vi "Keithley 2600 Series Merge.vi"() -> ()   [LabVIEW 2017]
doc: "This example shows how to create, run a script and query the script output data."
uses:
  <vilib>/Utility/file.llb/Write Delimited Spreadsheet (string).vi
  <instrlib>/Keithley 2600 Series/Keithley 2600 Series.lvlib
panel:
  in  "Yes":bool
  out "Continue":bool
  out "PCE(a.u.)":dbl
  in  "Pin(W/cm^2)":dbl=0.1
  out "FF(a.u.)":dbl
  out "Jsc(A/cm^2)":dbl
  in  "Area(cm^2)":dbl=0.085
  out "Ioc(A)":dbl
  out "Voc(V)":dbl
  out "Vsc(V)":dbl
  out "Isc(A)":dbl
  out "IMP(A)":dbl
  out "VMP(V)":dbl
  out "PMP(W)":dbl
  out "output array":string[][](array[string])
  in  "SweepSetting":T1={"CurrentLimit(A)"=0.1, "Start Voltage(V)"=-0.5, "Stop Voltage(V)"=0.9, "Dwell Time(mS)"=150.0, "NumPoint"=75.0} {"NumPoint" min=1.0 max=75.0 step=1.0; "Dwell Time(mS)" min=50.0 max=150.0; "Stop Voltage(V)" min=-200.0 max=200.0; "Start Voltage(V)" min=-200.0 max=200.0; "CurrentLimit(A)" min=1e-09 max=1.5}
  out "Graph 2":cluster{"Y":dbl[], "Y":dbl[]}[](graph)
  out "Sweep":i32
  in  "Inter Sweep Delay(s)":dbl=1.0 min=0.1 max=3600.0
  out "Seconds":i32
  out "Minutes":i32
  out "Hours":i32
  in  "Stop Button":bool
  in  "Aperture State (Channel B)":u16(ring) items=["Always OFF", "Always ON", "ON During Sweep OFF Otherwise", "OFF During Sweep ON Otherwise"]
  in  "Number of Sweeps":dbl=3.0 min=1.0 max=1000.0 step=1.0
  out "Working Folder":path
  in  "Folder Name":string="Raw Measurement"
  in  "USB COM Port":refnum<visa-resource-name>="COM3"
  # "Sweep Setting\n(Channel A)"
  # "Time Remaining"
  # ":"
  # ":"
  # "2634B can output up to 20.2 V at 1.5 A,\n or 202 V at 100 mA current limit."
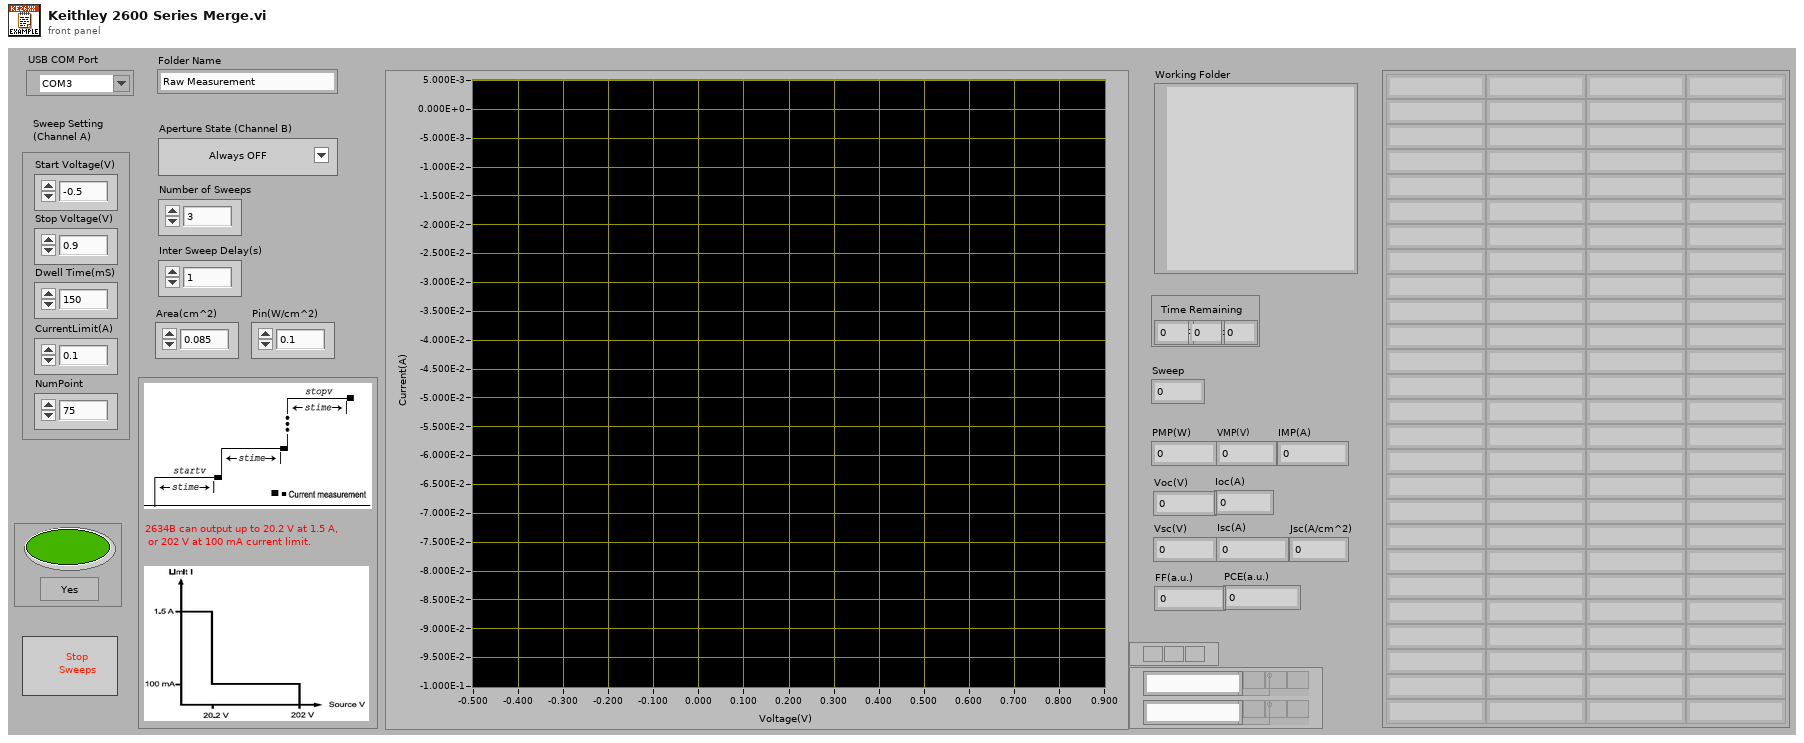
[diagram p1: front panel]
types:
  T1 = cluster{"CurrentLimit(A)":dbl, "Start Voltage(V)":dbl, "Stop Voltage(V)":dbl, "Dwell Time(mS)":dbl, "NumPoint":dbl}
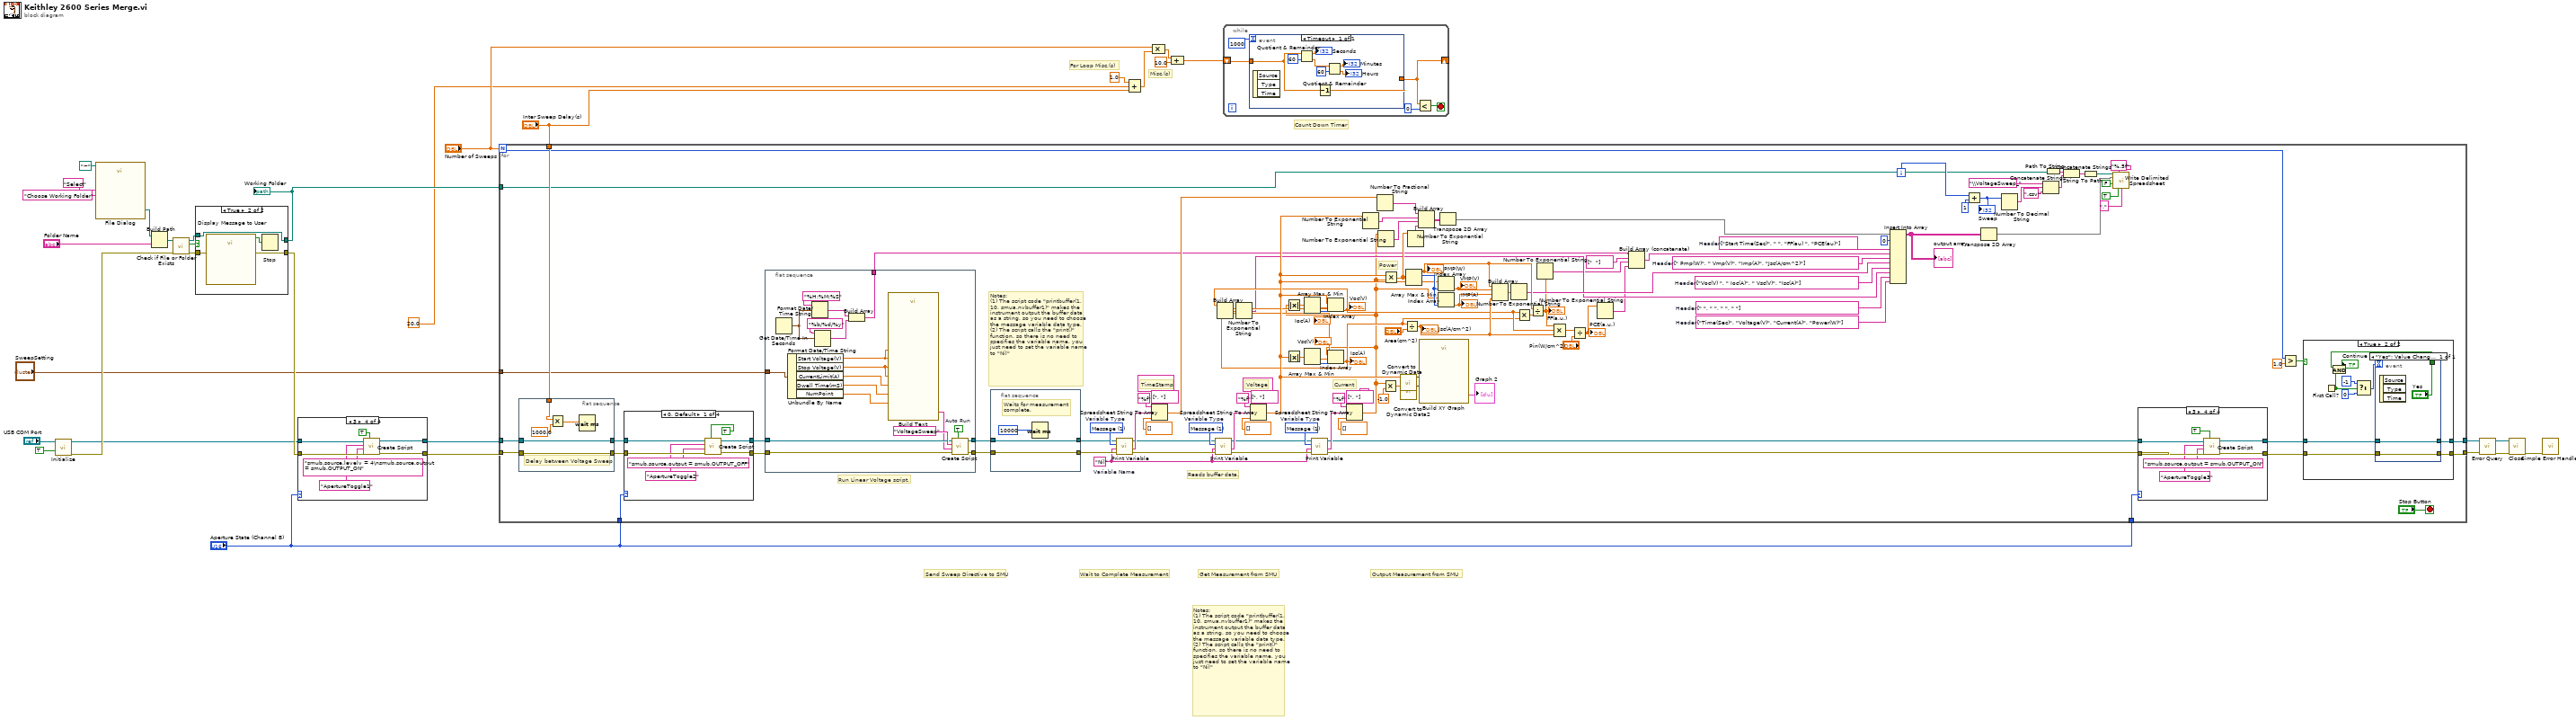
[diagram p0: block diagram]
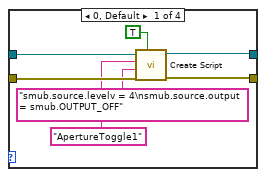
[diagram p2: hidden frame]
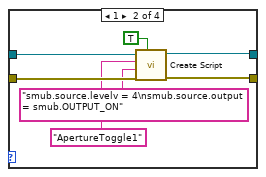
[diagram p3: hidden frame]
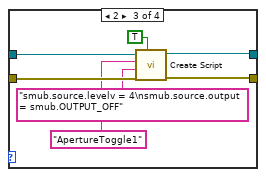
[diagram p4: hidden frame]
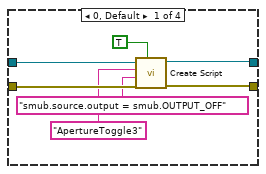
[diagram p6: hidden frame]
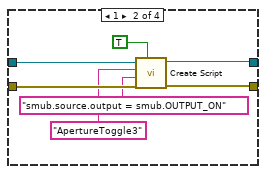
[diagram p7: hidden frame]
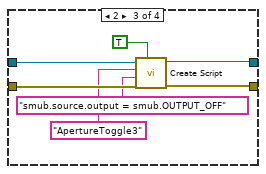
[diagram p8: hidden frame]
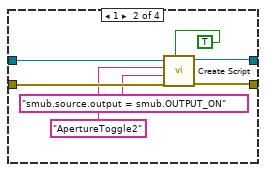
[diagram p9: hidden frame]
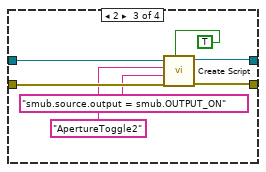
[diagram p10: hidden frame]
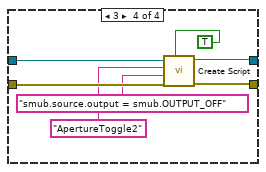
[diagram p11: hidden frame]
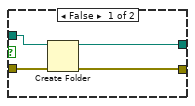
[diagram p12: hidden frame]
diagram:
  # "Count Down Timer"
  # "Misc.(s)"
  # "For Loop Misc.(s)"
  # "Send Sweep Directive to SMU"
  # "Wait to Complete Measurement"
  # "Output Measurement from SMU"
  # "Get Measurement from SMU"
  # "Notes: \n(1) The script code \"printbuffer(1, 10, smua.nvbuffer1)\" makes the instrument output the buffer data as a string, so you need to choose the message variable data type.\n(2) The script calls the \"print()\" function, so there is no need to specifies the variable name, you just need to set the variable name to \"Nil\""
  n1 = call <instrlib>:"Initialize.vi"("Reset (True)"=TRUE, "VISA resource name"="USB COM Port") -> ("error out"=w23:errorcluster, "VISA resource name out"=w16:refnum<visa-resource-name>)  [unwired: 8 in]
  n2 = call "File Dialog"("start path"=path "~", "prompt"="Choose Working Folder", "button label"="Select") -> ("selected path"=w5:path)  [unwired: 9 in, 3 out]
  n3 = Build Path(base path=w5, name or relative path="Folder Name") -> (appended path=w27:path)
  n4 = call <vilib>:"Check if File or Folder Exists.vi"("error in (no error)"=w23, "path"=w27) -> ("error out"=w24:errorcluster, "file or folder exists?"=w26:bool, "dup path"=w25:path)  [unwired: 7 in]
  n5 = case shown="True" w26 {
    tunnel: [w35 w38] -> w22
    tunnel: w25 -> [w36 w38]
    tunnel: w24 -> [w34 w40]
    tunnel: [w33 w37] -> w17
    frame False {
      n6 = Create Folder(path (use dialog)=w36, error in=w34) -> (created path=w35:path, error out=w33:errorcluster)  [unwired: 1 in, 1 out]
    }
    frame True {
      n7 = call "Display Message to User"("error in (no error)"=w40) -> ("error out"=w37:errorcluster, "OK"=w39:bool)  [unwired: 9 in]
      n8 = Stop(stop? (T)=w39) -> ()
    }
  }
  "Working Folder" <- w22
  n9 = case shown="3" "Aperture State (Channel B)" {
    tunnel: w16 -> [w47 w54 w61 w68]
    tunnel: w17 -> [w44 w51 w58 w65]
    tunnel: [w46 w53 w60 w67] -> w19
    tunnel: [w45 w52 w59 w66] -> w18
    frame 0, Default {
      n10 = call <instrlib>:"Create Script.vi"("Auto Run (F: Disable)"=TRUE, "error in (no error)"=w44, "Source Code"="smub.source.levelv = 4\nsmub.source.output = smub.OUTPUT_OFF", "Script Variable"="ApertureToggle1", "VISA resource name"=w47) -> ("error out"=w45:errorcluster, "VISA resource name out"=w46:refnum<visa-resource-name>)  [unwired: 5 in]
    }
    frame 1 {
      n11 = call <instrlib>:"Create Script.vi"("Auto Run (F: Disable)"=TRUE, "error in (no error)"=w51, "Source Code"="smub.source.levelv = 4\nsmub.source.output = smub.OUTPUT_ON", "Script Variable"="ApertureToggle1", "VISA resource name"=w54) -> ("error out"=w52:errorcluster, "VISA resource name out"=w53:refnum<visa-resource-name>)  [unwired: 5 in]
    }
    frame 2 {
      n12 = call <instrlib>:"Create Script.vi"("Auto Run (F: Disable)"=TRUE, "error in (no error)"=w58, "Source Code"="smub.source.levelv = 4\nsmub.source.output = smub.OUTPUT_OFF", "Script Variable"="ApertureToggle1", "VISA resource name"=w61) -> ("error out"=w59:errorcluster, "VISA resource name out"=w60:refnum<visa-resource-name>)  [unwired: 5 in]
    }
    frame 3 {
      n13 = call <instrlib>:"Create Script.vi"("Auto Run (F: Disable)"=TRUE, "error in (no error)"=w65, "Source Code"="smub.source.levelv = 4\nsmub.source.output = smub.OUTPUT_ON", "Script Variable"="ApertureToggle1", "VISA resource name"=w68) -> ("error out"=w66:errorcluster, "VISA resource name out"=w67:refnum<visa-resource-name>)  [unwired: 5 in]
    }
  }
  n14 = for {
    N: "Number of Sweeps" -> [w75]
    tunnel: w22 -> [w87]
    tunnel: "Aperture State (Channel B)" -> [w174]
    tunnel: "Aperture State (Channel B)" -> [w173]
    tunnel: "Inter Sweep Delay(s)" -> [w172]
    tunnel: "SweepSetting" -> [w85]
    tunnel: w19 -> [w178]
    tunnel: [w70] -> w21
    tunnel: w18 -> [w177]
    tunnel: [w71] -> w20
    i -> [w158]
    stop <- "Stop Button" stop-if-true
    w95 = string[] ["Voc(V) ", " Ioc(A)", " Vsc(V)", "Isc(A)"]  # Header
    w96 = string[] [" Pmp(W)", " Vmp(V)", "Imp(A)", "Jsc(A/cm^2)"]  # Header
    w92 = string[] ["Time(Sec)", "Voltage(V)", "Current(A)", "Power(W)"]  # Header
    w93 = string[] [" ", " ", " ", " "]  # Header
    w109 = string[] ["Start Time(Sec)", " ", "FF(au) ", "PCE(au)"]  # Header
    w142 = 1 items=["Number", "Message"]  # Variable Type
    w143 = 1 items=["Number", "Message"]  # Variable Type
    w157 = 1 items=["Number", "Message"]  # Variable Type
    w133 = "Nil"  # Variable Name
    # "Power"
    # "Current"
    # "Voltage"
    # "TimeStamp"
    # "Reads buffer data."
    # "Notes: \n(1) The script code \"printbuffer(1, 10, smua.nvbuffer1)\" makes the instrument output the buffer data as a string, so you need to choose the message variable data type.\n(2) The script calls the \"print()\" function, so there is no need to specifies the variable name, you just need to set the variable name to \"Nil\""
    # "Run Linear Voltage script."
    n15 = flat-sequence {
      tunnel: w178 -> [w276]
      tunnel: w177 -> [w275]
      tunnel: [w276] -> w176
      tunnel: [w275] -> w175
      tunnel: w172 -> [w272]
      frame #0 {
        # "Delay between Voltage Sweep"
        n16 = Multiply(x=w272, y=1000.0) -> (x*y=w274:dbl)
        n17 = Wait (ms)(milliseconds to wait=w274) -> ()  [unwired: 1 out]
      }
    }
    n18 = case shown="0, Default" w174 {
      tunnel: w176 -> [w250 w257 w264 w271]
      tunnel: w175 -> [w247 w254 w261 w268]
      tunnel: [w249 w256 w263 w270] -> w91
      tunnel: [w248 w255 w262 w269] -> w90
      frame 0, Default {
        n19 = call <instrlib>:"Create Script.vi"("Auto Run (F: Disable)"=TRUE, "error in (no error)"=w247, "Source Code"="smub.source.output = smub.OUTPUT_OFF", "Script Variable"="ApertureToggle2", "VISA resource name"=w250) -> ("error out"=w248:errorcluster, "VISA resource name out"=w249:refnum<visa-resource-name>)  [unwired: 5 in]
      }
      frame 1 {
        n20 = call <instrlib>:"Create Script.vi"("Auto Run (F: Disable)"=TRUE, "error in (no error)"=w254, "Source Code"="smub.source.output = smub.OUTPUT_ON", "Script Variable"="ApertureToggle2", "VISA resource name"=w257) -> ("error out"=w255:errorcluster, "VISA resource name out"=w256:refnum<visa-resource-name>)  [unwired: 5 in]
      }
      frame 2 {
        n21 = call <instrlib>:"Create Script.vi"("Auto Run (F: Disable)"=TRUE, "error in (no error)"=w261, "Source Code"="smub.source.output = smub.OUTPUT_ON", "Script Variable"="ApertureToggle2", "VISA resource name"=w264) -> ("error out"=w262:errorcluster, "VISA resource name out"=w263:refnum<visa-resource-name>)  [unwired: 5 in]
      }
      frame 3 {
        n22 = call <instrlib>:"Create Script.vi"("Auto Run (F: Disable)"=TRUE, "error in (no error)"=w268, "Source Code"="smub.source.output = smub.OUTPUT_OFF", "Script Variable"="ApertureToggle2", "VISA resource name"=w271) -> ("error out"=w269:errorcluster, "VISA resource name out"=w270:refnum<visa-resource-name>)  [unwired: 5 in]
      }
    }
    n23 = flat-sequence {
      tunnel: [w210] -> w156
      tunnel: [w209] -> w155
      tunnel: w91 -> [w208]
      tunnel: w90 -> [w207]
      tunnel: [w200] -> w111
      tunnel: w85 -> [w194]
      frame #0 {
        w211 = TRUE  # Auto Run
        n24 = Get Date/Time In Seconds() -> (seconds since 1Jan1904=w201:timestamp)
        n25 = Unbundle By Name(w194) -> ("Start Voltage(V)"=w199:dbl, "Stop Voltage(V)"=w198:dbl, "CurrentLimit(A)"=w197:dbl, "Dwell Time(mS)"=w196:dbl, "NumPoint"=w195:dbl)
        n26 = Format Date/Time String(time format string (%c)="%H:%M:%S", seconds (now)=w201) -> (date/time string=w204:string)  [unwired: 1 out]
        n27 = Format Date/Time String(time format string (%c)="%b/%d/%y", seconds (now)=w201) -> (date/time string=w202:string)  [unwired: 1 out]
        n28 = Build Array(w204, w202) -> (w200:string[])
        n29 = call "Build Text"("numPoints"=w195, "stopV1"=w198, "limitI"=w197, "stopV"=w198, "startV"=w199, "startV1"=w199, "dwellTime"=w196) -> ("Result"=w206:string)  [unwired: 7 in, 1 out]
        n30 = call <instrlib>:"Create Script.vi"("Auto Run (F: Disable)"=w211, "error in (no error)"=w207, "Source Code"=w206, "Script Variable"="VoltageSweep" ("Script Variable (myScript)"), "VISA resource name"=w208) -> ("error out"=w209:errorcluster, "VISA resource name out"=w210:refnum<visa-resource-name>)  [unwired: 5 in]
      }
    }
    n31 = flat-sequence {
      tunnel: w156 -> [w213]
      tunnel: w155 -> [w214]
      tunnel: [w214] -> w153
      tunnel: [w213] -> w154
      frame #0 {
        # "Waits for measurement complete."
        n32 = Wait (ms)(milliseconds to wait=10000 ("Temp Delay")) -> ()  [unwired: 1 out]
      }
    }
    n33 = call <instrlib>:"Print Variable.vi"("error in (no error)"=w153, "Variable Name"=w133, "Variable Type (0: Number)"=w157, "VISA resource name"=w154) -> ("error out"=w139:errorcluster, "Message"=w148:string, "VISA resource name out"=w140:refnum<visa-resource-name>)  [unwired: 4 in, 1 out]
    n34 = Spreadsheet String To Array(delimiter (Tab)=string[] [", "], format string="%f", spreadsheet string=w148, array type (2D Dbl)=dbl[] []) -> (array=w128:dbl[])
    n35 = call <instrlib>:"Print Variable.vi"("error in (no error)"=w139, "Variable Name"=w133, "Variable Type (0: Number)"=w143, "VISA resource name"=w140) -> ("error out"=w137:errorcluster, "Message"=w147:string, "VISA resource name out"=w138:refnum<visa-resource-name>)  [unwired: 4 in, 1 out]
    n36 = Spreadsheet String To Array(delimiter (Tab)=string[] [", "], format string="%f", spreadsheet string=w147, array type (2D Dbl)=dbl[] []) -> (array=w118:dbl[])
    n37 = Absolute Value(x=w118) -> (abs(x)=w122:dbl[])
    n38 = Array Max & Min(array=w122) -> (min value=w98:dbl, min index (indices)=w121:i32)  [unwired: 2 out]
    "Vsc(V)" <- w98
    n39 = call <instrlib>:"Print Variable.vi"("error in (no error)"=w137, "Variable Name"=w133, "Variable Type (0: Number)"=w142, "VISA resource name"=w138) -> ("error out"=w88:errorcluster, "Message"=w135:string, "VISA resource name out"=w89:refnum<visa-resource-name>)  [unwired: 4 in, 1 out]
    n40 = Spreadsheet String To Array(delimiter (Tab)=string[] [", "], format string="%f", spreadsheet string=w135, array type (2D Dbl)=dbl[] []) -> (array=w78:dbl[])
    n41 = Absolute Value(x=w78) -> (abs(x)=w119:dbl[])
    n42 = Array Max & Min(array=w119) -> (min value=w99:dbl, min index (indices)=w120:i32)  [unwired: 2 out]
    "Ioc(A)" <- w99
    n43 = Index Array(array=w118, index=w120) -> (element=w100:dbl)
    "Voc(V)" <- w100
    n44 = Index Array(array=w78, index=w121) -> (element=w97:dbl)
    "Isc(A)" <- w97
    n45 = Build Array(w100, w99, w98, w97) -> (w101:dbl[])
    n46 = Number To Exponential String(number=w101) -> (E-format string=w94:string[])  [unwired: 3 in]
    n47 = Number To Exponential String(number=w118) -> (E-format string=w130:string[])  [unwired: 3 in]
    n48 = Number To Fractional String(number=w128) -> (F-format string=w131:string[])  [unwired: 3 in]
    n49 = Number To Exponential String(number=w78) -> (E-format string=w126:string[])  [unwired: 3 in]
    n50 = Multiply(x=w78, y=-1.0) -> (x*y=w80:dbl[])
    n51 = Multiply(x=w118, y=w78) -> (x*y=w112:dbl[])
    n52 = call "Convert to Dynamic Data"("Array"=w118) -> ("Dynamic Data Type"=w125:dynamicdata)  [unwired: 3 in]
    n53 = call "Convert to Dynamic Data2"("Array"=w80) -> ("Dynamic Data Type"=w124:dynamicdata)  [unwired: 3 in]
    n54 = Divide(x=w97, y="Area(cm^2)") -> (x/y=w104:dbl)
    "Jsc(A/cm^2)" <- w104
    n55 = Array Max & Min(array=w112) -> (max value=w107:dbl, max index (indices)=w123:i32)  [unwired: 2 out]
    "PMP(W)" <- w107
    n56 = Number To Exponential String(number=w112) -> (E-format string=w113:string[])  [unwired: 3 in]
    n57 = Build Array(w131, w130, w126, w113) -> (w132:string[][])
    n58 = call "Build XY Graph"("Y Input"=w124, "X Input"=w125) -> ("XY Graph"=→"Graph 2":cluster{"X":dbl[], "Y":dbl[]}[])  [unwired: 8 in, 1 out]
    n59 = Index Array(array=w118, index=w123) -> (element=w106:dbl)
    "VMP(V)" <- w106
    n60 = Index Array(array=w78, index=w123) -> (element=w105:dbl)
    "IMP(A)" <- w105
    n61 = Transpose 2D Array(2D array=w132) -> (transposed array=w129:string[][])
    n62 = Build Array(w107, w106, w105, w104) -> (w103:dbl[])
    n63 = Number To Exponential String(number=w103) -> (E-format string=w102:string[])  [unwired: 3 in]
    n64 = Multiply(x=w97, y=w100) -> (x*y=w116:dbl)
    n65 = Divide(x=w107, y=w116) -> (x/y=w84:dbl)
    "FF(a.u.)" <- w84
    n66 = Number To Exponential String(number=w84) -> (E-format string=w83:string)  [unwired: 3 in]
    n67 = Compound Arithmetic op=MULTIPLY(w84, w100, w104) -> (w115:dbl)
    n68 = Divide(x=w115, y="Pin(W/cm^2)") -> (x/y=w82:dbl)
    "PCE(a.u.)" <- w82
    n69 = Number To Exponential String(number=w82) -> (E-format string=w81:string)  [unwired: 3 in]
    n70 = Build Array (concatenate)(w111, string[] ["  "] ("element"), w83, w81) -> (w108:string[])
    n71 = Insert Into Array(array=w129, index (row)=0, new element #1=w109, new element #2=w108, new element #3=w96, new element #4=w102, new element #5=w95, new element #6=w94, new element #7=w93, new element #8=w92) -> (w86:string[][])  [unwired: 1 in]
    "output array" <- w86
    n72 = Add(x=w158, y=1 ("x")) -> (x+y=w171:i32)
    "Sweep" <- w171
    n73 = Transpose 2D Array(2D array=w86) -> (transposed array=w77:string[][])
    n74 = Number To Decimal String(number=w171) -> (decimal integer string=w170:string)  [unwired: 1 in]
    n75 = Concatenate Strings("\\VoltageSweep_" ("string"), w170, ".csv" ("string")) -> (w169:string)
    n76 = Path To String(path=w87) -> (string=w166:string)
    n77 = Concatenate Strings(w166, w169) -> (w167:string)
    n78 = String To Path(string=w167) -> (path=w168:path)
    n79 = call-poly <vilib>:"Write Delimited Spreadsheet.vi"("file path (dialog if empty)"=w168, "format (%s)"="%.5f" ("format (%.3f)"), "2D data"=w77, "append to file? (new file:F)"=FALSE, "transpose? (no:F)"=TRUE, "delimiter (\\t)"="," ("delimiter (\\t)")) -> ()  [unwired: 8 in, 2 out]
    n80 = case shown="3" w173 {
      tunnel: w89 -> [w222 w229 w236 w243]
      tunnel: w88 -> [w219 w226 w233 w240]
      tunnel: [w221 w228 w235 w242] -> w73
      tunnel: [w220 w227 w234 w241] -> w72
      frame 0, Default {
        n81 = call <instrlib>:"Create Script.vi"("Auto Run (F: Disable)"=TRUE, "error in (no error)"=w219, "Source Code"="smub.source.output = smub.OUTPUT_OFF", "Script Variable"="ApertureToggle3", "VISA resource name"=w222) -> ("error out"=w220:errorcluster, "VISA resource name out"=w221:refnum<visa-resource-name>)  [unwired: 5 in]
      }
      frame 1 {
        n82 = call <instrlib>:"Create Script.vi"("Auto Run (F: Disable)"=TRUE, "error in (no error)"=w226, "Source Code"="smub.source.output = smub.OUTPUT_ON", "Script Variable"="ApertureToggle3", "VISA resource name"=w229) -> ("error out"=w227:errorcluster, "VISA resource name out"=w228:refnum<visa-resource-name>)  [unwired: 5 in]
      }
      frame 2 {
        n83 = call <instrlib>:"Create Script.vi"("Auto Run (F: Disable)"=TRUE, "error in (no error)"=w233, "Source Code"="smub.source.output = smub.OUTPUT_OFF", "Script Variable"="ApertureToggle3", "VISA resource name"=w236) -> ("error out"=w234:errorcluster, "VISA resource name out"=w235:refnum<visa-resource-name>)  [unwired: 5 in]
      }
      frame 3 {
        n84 = call <instrlib>:"Create Script.vi"("Auto Run (F: Disable)"=TRUE, "error in (no error)"=w240, "Source Code"="smub.source.output = smub.OUTPUT_ON", "Script Variable"="ApertureToggle3", "VISA resource name"=w243) -> ("error out"=w241:errorcluster, "VISA resource name out"=w242:refnum<visa-resource-name>)  [unwired: 5 in]
      }
    }
    n85 = Greater?(x=w75, y=1.0) -> (0:w69:bool)
    n86 = case shown="True" w69 {
      tunnel: w73 -> [w180 w186]
      tunnel: w72 -> [w179 w185]
      tunnel: [w179 w184] -> w71
      tunnel: [w180 w183] -> w70
      frame False {
      }
      frame True {
        n87 = First Call?() -> (First Call?: T/F=w187:bool)
        n88 = Select(t=-1, s=w187, f=0) -> (s? t:f=w190:i32)
        n89 = event shown="[0] \"Yes\": Value Change;  Timeout" {
          selector: _ -> [_]
          dyn-events: _ -> [_]
          timeout: w190 -> [_]
          tunnel: w186 -> [w193]
          tunnel: w185 -> [w192]
          tunnel: [w193] -> w183
          tunnel: [w192] -> w184
          tunnel: ["Yes"] -> w181
          event "Yes": Value Change; Timeout {
            n90 = event-data() -> ()  [unwired: 1 in, 3 out]
          }
        }
        n91 = And(x=w181, y=w187) -> (x .and. y?=→"Continue":bool)
      }
    }
  }
  n92 = Compound Arithmetic op=ADD(1.0 ("value"), 20.0 ("value"), "Inter Sweep Delay(s)") -> (w13:dbl)
  n93 = Compound Arithmetic op=MULTIPLY("Number of Sweeps", w13) -> (w12:dbl)
  n94 = Compound Arithmetic op=ADD(w12, 10.0 ("value")) -> (w10:dbl)
  n95 = while {
    shift-right: [w278] -> _
    shift-left: w10 -> [w280]
    stop <- w279 stop-if-true
    n96 = event shown="[0] Timeout" {
      selector: _ -> [_]
      dyn-events: _ -> [_]
      timeout: 1000 -> [_]
      tunnel: w280 -> [w287]
      tunnel: [w289] -> w278
      event Timeout {
        n97 = event-data() -> ()  [unwired: 1 in, 3 out]
        n98 = Quotient & Remainder(x=w287, y=60) -> (x-y*floor(x/y)=→"Seconds":dbl, floor(x/y)=w283:dbl)
        n99 = Decrement(x=w287) -> (x-1=w289:dbl)
        n100 = Quotient & Remainder(x=w283, y=60) -> (x-y*floor(x/y)=→"Minutes":dbl, floor(x/y)=→"Hours":dbl)
      }
    }
    n101 = Less?(x=w278, y=0) -> (x < y?=w279:bool)
  }
  n102 = call <instrlib>:"Error Query.vi"("error in (no error)"=w20, "VISA resource name"=w21) -> ("error out"=w31:errorcluster, "VISA resource name out"=w32:refnum<visa-resource-name>)  [unwired: 6 in, 2 out]
  n103 = call <instrlib>:"Close.vi"("error in (no error)"=w31, "VISA resource name"=w32) -> ("error out"=w2:errorcluster)  [unwired: 9 in]
  n104 = call <vilib>:"Simple Error Handler.vi"("error in (no error)"=w2) -> ()  [unwired: 4 in, 5 out]
